vi "RTFlipMirror.vi"(8 "error in (no error)":errorcluster) -> (0 "error out":errorcluster)   [LabVIEW 2016]
uses:
  Classes/FlipMir/Flip Mirror Containter.lvclass
  Controls/Operational Modes.ctl
  Controls/Flip Mirrors.ctl
  Controls/Mirror Data.ctl
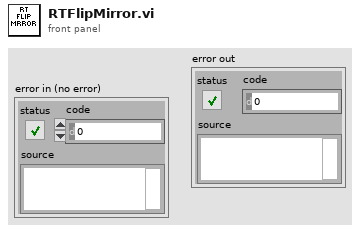
[diagram p1: front panel]
types:
  T1 = typedef "Operational Modes.ctl" = enum16{"Sci", "Sci-LFC", "Solar", "Solar-LFC", "LFC", "LFC-Sim", "LFC-Both", "ThAr", "ThAr-LFC", "Flat", "ExtFlat", "ExtFlat-Sim", "ExtFlat-Both", "Qtz", "ExtQtz", "ExtQtz-Sim", "ExtQtz-Both", "Dark", "Manual", "Off"}
  T2 = typedef "Flip Mirrors.ctl" = cluster{"ExtFlat":T3, "ThAr":T3, "Solar":T3}
  T3 = typedef "Mirror Data.ctl" = cluster{"Status":bool, "Time Stamp":timestamp}
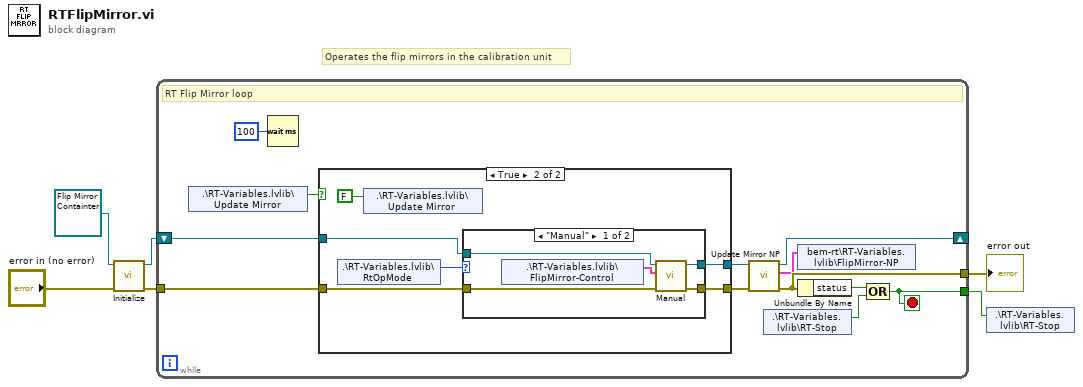
[diagram p0: block diagram]
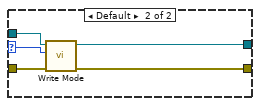
[diagram p3: hidden frame]
diagram:
  # "Operates the flip mirrors in the calibration unit"
  n1 = call-dynamic "Initialize.vi"("error in (no error)"="error in (no error)", "Flip Mirror Containter in"=refnum<class "Flip Mirror Containter.lvclass"> refnum ("Flip Mirror Containter.lvclass")) -> ("error out"=w5:errorcluster, "Flip Mirror Containter out"=w4:refnum<class "Flip Mirror Containter.lvclass">)  [unwired: 8 in]
  n2 = while {
    tunnel: w5 -> [w9]
    tunnel: [w16] -> w6
    tunnel: [w15] -> w1
    shift-right: [w13] -> _
    shift-left: w4 -> [w11]
    stop <- w16 stop-if-true
    # "RT Flip Mirror loop"
    n3 = shared-variable ".\\RT-Variables.lvlib\\Update Mirror"() -> (w18:bool)  [unwired: 1 in, 1 out]
    n4 = Wait (ms)(milliseconds to wait=u32 100) -> ()  [unwired: 1 out]
    n5 = case shown="True" w18 {
      tunnel: w11 -> [w20 w24]
      tunnel: [w20 w22] -> w10
      tunnel: w9 -> [w19 w23]
      tunnel: [w19 w21] -> w8
      frame False {
      }
      frame True {
        n6 = shared-variable ".\\RT-Variables.lvlib\\RtOpMode"() -> (w26:T1)  [unwired: 1 in, 1 out]
        n7 = shared-variable ".\\RT-Variables.lvlib\\Update Mirror"(FALSE ("Update Mirror")) -> ()  [unwired: 1 in, 1 out]
        n8 = case shown="\"Manual\"" w26 {
          selector: w26 -> [_ w34]
          tunnel: w24 -> [w31 w36]
          tunnel: w23 -> [w30 w35]
          tunnel: [w29 w33] -> w22
          tunnel: [w28 w32] -> w21
          frame "Manual" {
            n9 = shared-variable ".\\RT-Variables.lvlib\\FlipMirror-Control"() -> (w27:T2)  [unwired: 1 in, 1 out]
            n10 = call-dynamic "Manual.vi"("error in (no error)"=w30, "Mirrors"=w27, "Flip Mirror Containter in"=w31) -> ("error out"=w28:errorcluster, "Flip Mirror Containter out"=w29:refnum<class "Flip Mirror Containter.lvclass">)  [unwired: 7 in]
          }
          frame Default {
            n11 = call-dynamic "Write Mode.vi"("error in (no error)"=w35, "Operational Mode"=w34, "Flip Mirror Containter in"=w36) -> ("error out"=w32:errorcluster, "Flip Mirror Containter out"=w33:refnum<class "Flip Mirror Containter.lvclass">)  [unwired: 7 in]
          }
        }
      }
    }
    n12 = call "Update Mirror NP.vi"("error in (no error)"=w8, "Flip Mirror Containter in"=w10) -> ("error out"=w15:errorcluster, "Mirrors-NP"=w12:T2, "Flip Mirror Containter out"=w13:refnum<class "Flip Mirror Containter.lvclass">)  [unwired: 7 in]
    n13 = shared-variable ".\\RT-Variables.lvlib\\RT-Stop"() -> (w17:bool)  [unwired: 1 in, 1 out]
    n14 = shared-variable "bem-rt\\RT-Variables.lvlib\\FlipMirror-NP"(w12) -> ()  [unwired: 1 in, 1 out]
    n15 = Unbundle By Name(w15) -> ("status"=w14:bool)
    n16 = Compound Arithmetic op=OR(w14, w17) -> (w16:bool)
  }
  "error out" <- w1
  n17 = shared-variable ".\\RT-Variables.lvlib\\RT-Stop"(w6) -> ()  [unwired: 1 in, 1 out]
